vi "AutoMode.vi"   [LabVIEW 2024]
uses:
  DataTypes/OperationTypeForFunctionalGlobalVariable.ctl
types:
  T1 = typedef "OperationTypeForFunctionalGlobalVariable.ctl" = enum16{"GET", "SET"}
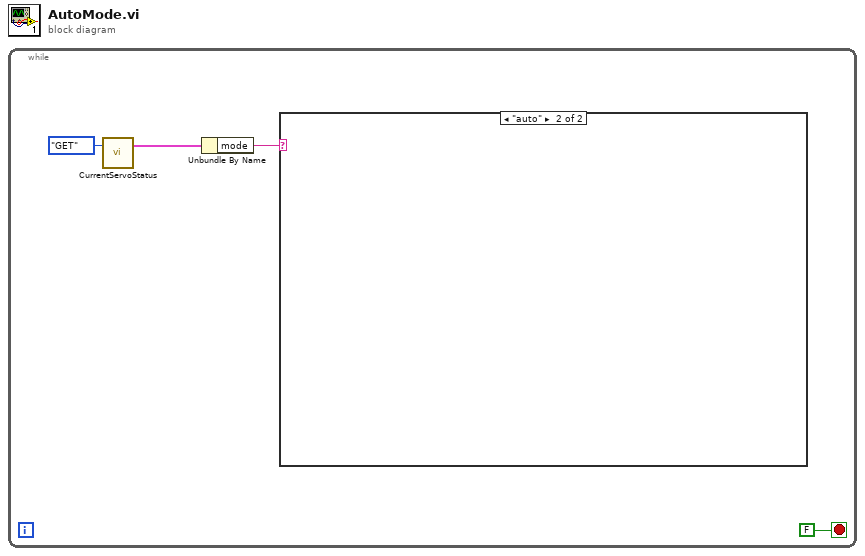
[diagram p0: block diagram]
diagram:
  n1 = while {
    stop <- FALSE stop-if-true
    n2 = call "CurrentServoStatus.vi"("Operation"=OperationTypeForFunctionalGlobalVariable."GET") -> ("Current Servo Status"=w2:cluster{"mode":string, "position":dbl})  [unwired: 2 in]
    n3 = Unbundle By Name(w2) -> ("mode"=w1:string)
    n4 = case shown="\"auto\"" w1 {
      frame "manual", Default {
      }
      frame "auto" {
      }
    }
  }
